vi "String - Create DAT File Header.vi"(11 "Channel to Probe Mapping":string) -> (2 ".dat Header":string, 3 "Valid Channel List":string[](array[string]))   [LabVIEW 2013]
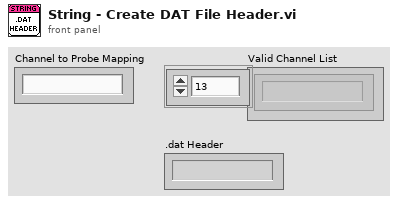
[diagram p1: front panel]
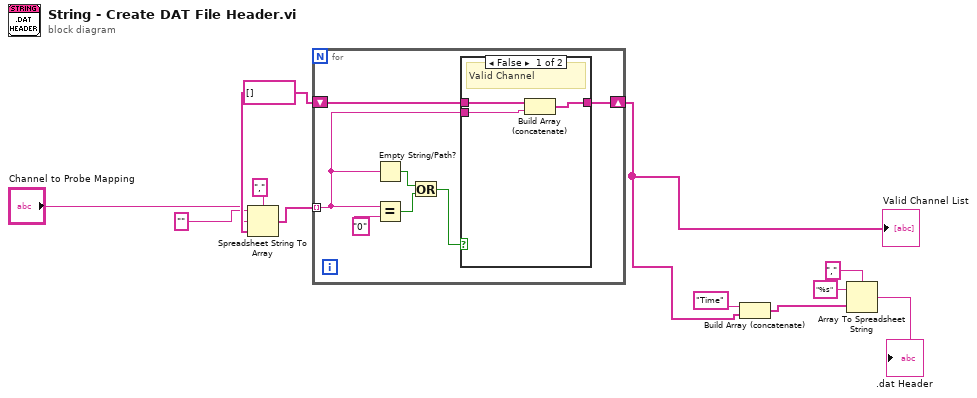
[diagram p0: block diagram]
diagram:
  w8 = string[] []
  n1 = Spreadsheet String To Array(delimiter (Tab)=",", format string="", spreadsheet string="Channel to Probe Mapping", array type (2D Dbl)=w8) -> (array=w9:string[])
  n2 = for {
    tunnel: w9 -> [w15] mode=indexing
    shift-right: [w17] -> w1
    shift-left: w8 -> [w18]
    n3 = Empty String/Path?(string/path=w15) -> (empty?=w14:bool)
    n4 = Equal?(x=w15, y="0") -> (x = y?=w13:bool)
    n5 = Or(x=w14, y=w13) -> (x .or. y?=w12:bool)
    n6 = case shown="False" w12 {
      tunnel: w18 -> [w21 w22]
      tunnel: w15 -> [w20 _]
      tunnel: [w19 w22] -> w17
      frame False {
        # "Valid Channel"
        n7 = Build Array (concatenate)(w21, w20) -> (w19:string[])
      }
      frame True {
        # "Blank or 0 - Skip"
      }
    }
  }
  "Valid Channel List" <- w1
  n8 = Build Array (concatenate)("Time", w1) -> (w11:string[])
  n9 = Array To Spreadsheet String(delimiter (Tab)=",", array=w11, 3:"%s" ("format string")) -> (spreadsheet string=→".dat Header":string)
